vi "Arduino.vi"(3 "Config Serial":T1={"Puerto Serial"="", "Baudios"=9600, "Data Bis"=8, "Paridad"=enum."None", "Bits Stop"=10, "Control"=0} {"Control" items=["None", "XON/XOFF", "RTS/CTS", "XON/XOFF & RTS/CTS", "DTR/DSR", "XON/XOFF & DTR/DSR"]; "Bits Stop" items=["1.0"=10, "1.5"=15, "2.0"=20]; "Data Bis" min=5 max=8 step=1}) -> ()   [LabVIEW 2020]
uses:
  <vilib>/Instr/_visa.llb/VISA Configure Serial Port (Instr).vi
  <vilib>/ErrorRing/Error Ring.xnode
panel:
  in  "Boolean 2":bool
  out "Boolean":bool
  out "RX":string
  in  "?":bool
  # "Comunicación Serial"
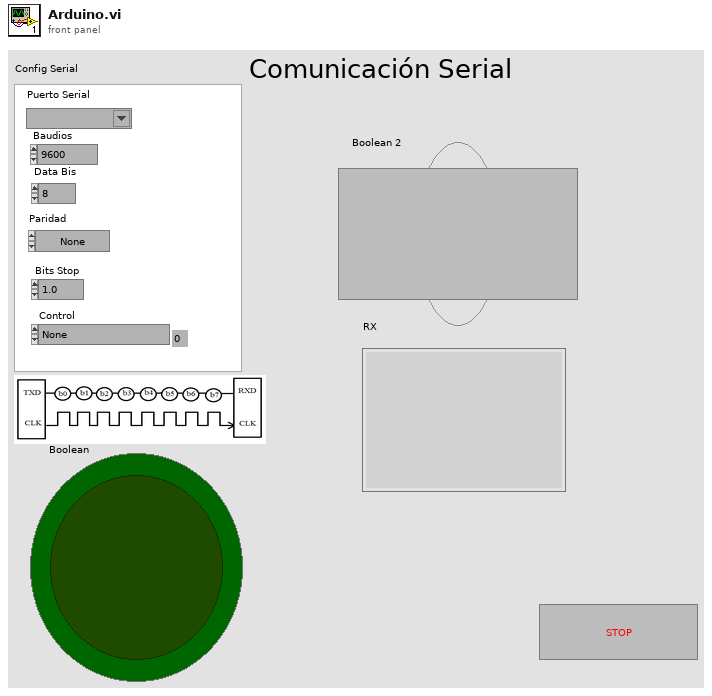
[diagram p1: front panel]
types:
  T1 = cluster{"Puerto Serial":refnum<visa-resource-name>, "Baudios":u32, "Data Bis":u16, "Paridad":enum16{"None", "Odd", "Even", "Mark", "Space"}, "Bits Stop":u16, "Control":u16}
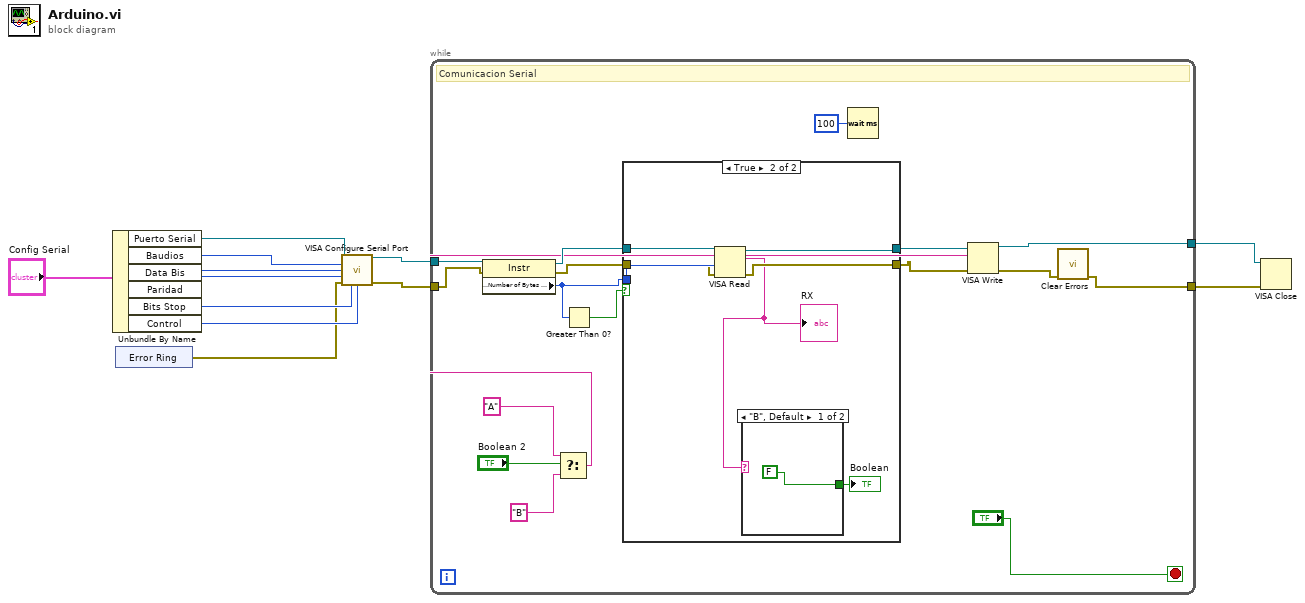
[diagram p0: block diagram]
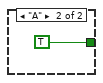
[diagram p3: hidden frame]
diagram:
  n1 = Unbundle By Name("Config Serial") -> ("Puerto Serial"=w11:refnum<visa-resource-name>, "Baudios"=w10:u32, "Data Bis"=w9:u16, "Paridad"=w8:enum16{"None", "Odd", "Even", "Mark", "Space"}, "Bits Stop"=w7:u16, "Control"=w6:u16)
  n2 = xnode "Error Ring"() -> ("error out"=w5:errorcluster)
  n3 = call-poly "VISA Configure Serial Port"("VISA resource name"=w11, "baud rate (9600)"=w10, "data bits (8)"=w9, "parity (0:none)"=w8, "error in (no error)"=w5, "stop bits (10: 1 bit)"=w7, "flow control (0:none)"=w6) -> ("VISA resource name out"=w4:refnum<visa-resource-name>, "error out"=w3:errorcluster)  [unwired: 7 in]
  n4 = while {
    tunnel: w4 -> [w24]
    tunnel: w3 -> [w23]
    tunnel: [w13] -> w2
    tunnel: [w15] -> w1
    stop <- "?" stop-if-true
    # "Comunicacion Serial"
    n5 = property class="Instr"(reference=w24, error in=w23) -> (reference out=w27:refnum<visa-resource-name>, error out=w26:errorcluster, "Serial Settings:Number of Bytes at Serial Port"=w25:u32)
    n6 = Select(t="A", s="Boolean 2", f="B") -> (s? t:f=w16:string)
    n7 = Greater Than 0?(x=w25) -> (x > 0?=w28:bool)
    n8 = case shown="True" w28 {
      tunnel: [w31 w34] -> w18
      tunnel: w27 -> [w31 w38]
      tunnel: w26 -> [w30 w36]
      tunnel: [w30 w35] -> w17
      tunnel: w25 -> [_ w37]
      frame False {
      }
      frame True {
        n9 = VISA Read(VISA resource name=w38, byte count=w37, error in (no error)=w36) -> (VISA resource name out=w34:refnum<visa-resource-name>, read buffer=w33:string, error out=w35:errorcluster)  [unwired: 1 out]
        "RX" <- w33
        n10 = case shown="\"B\", Default" w33 {
          tunnel: [FALSE TRUE] -> w32
          frame "B", Default {
          }
          frame "A" {
          }
        }
        "Boolean" <- w32
      }
    }
    n11 = Wait (ms)(milliseconds to wait=u32 100) -> ()  [unwired: 1 out]
    n12 = VISA Write(VISA resource name=w18, write buffer=w16, error in (no error)=w17) -> (VISA resource name out=w15:refnum<visa-resource-name>, error out=w14:errorcluster)  [unwired: 1 out]
    n13 = call <vilib>:"Clear Errors.vi"("error in (no error)"=w14) -> ("error out"=w13:errorcluster)  [unwired: 5 in, 1 out]
  }
  n14 = VISA Close(VISA resource name=w1, error in (no error)=w2) -> ()  [unwired: 1 out]
